vi "Config Types.vi"(8 "error in (no error)":errorcluster, 11 "Reconfigurable in":refnum<class "Reconfigurable.lvclass">) -> (0 "error out":errorcluster, 2 "Config Types":string[](array[string]), 3 "Reconfigurable out":refnum<class "Reconfigurable.lvclass">)   [LabVIEW 2020, in "Volatus.lvlib" / "Reconfigurable.lvclass"]
uses:
  Reconfigurable.lvclass
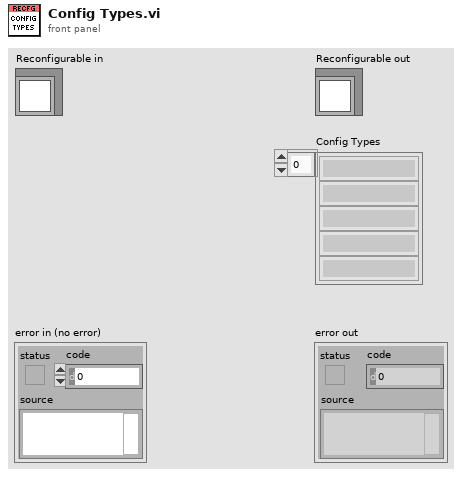
[diagram p1: front panel]
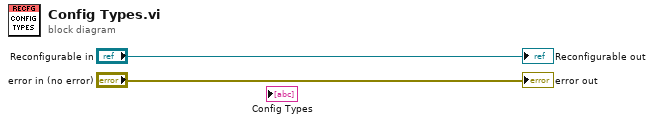
[diagram p0: block diagram]
diagram:
  "error out" <- "error in (no error)"
  "Reconfigurable out" <- "Reconfigurable in"
